vi "Marshal.vi"(8 "error in (no error)":errorcluster, 11 "int32 in":refnum<class "packed.lvclass">) -> (0 "error out":errorcluster, 2 "Buffer":u8[](array[numeric]), 3 "int32 out":refnum<class "packed.lvclass">)   [LabVIEW 2020, in "Protobuf RAW.lvlib" / "packed.lvclass"]
uses:
  packed.lvclass
  packed.lvclass/packed.ctl
  Scalar Encoder/Scalar Type.lvclass
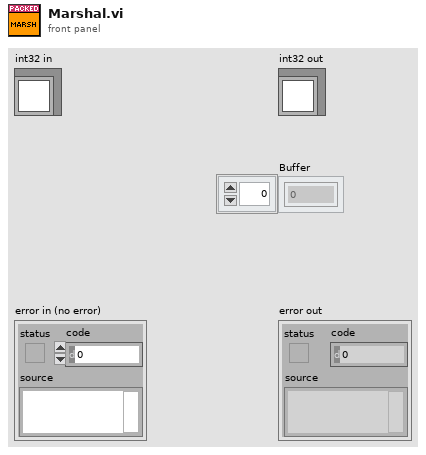
[diagram p1: front panel]
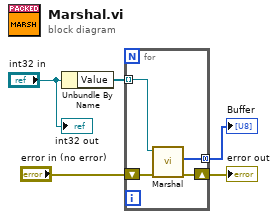
[diagram p0: block diagram]
diagram:
  n1 = Unbundle By Name("int32 in") -> ("Value"=w4:refnum<class "Scalar Type.lvclass">[])
  n2 = for {
    tunnel: w4 -> [w9] mode=indexing
    tunnel: [w8] -> w3 mode=concatenating
    shift-right: [w6] -> w1
    shift-left: "error in (no error)" -> [w7]
    n3 = call-dynamic "Marshal.vi"("error in (no error)"=w7, "Type Serializer in"=w9) -> ("error out"=w6:errorcluster, "Buffer"=w8:u8[])  [unwired: 7 in, 1 out]
  }
  "error out" <- w1
  "Buffer" <- w3
  "int32 out" <- "int32 in"
